vi "Initialize MeasurementLink Session.vi"(7 "remote connection options":T2, 8 "error in":errorcluster, 9 "initialize and close session behavior":T1, 10 "session initialization parameters":T3, 11 "session factory in":refnum<class "Session Factory.lvclass">) -> (0 "error out":errorcluster, 2 "session out":variant, 3 "session factory out":refnum<class "Session Factory.lvclass">)   [LabVIEW 2021, in "NI Session Management niDMM.lvlib" / "Session Factory.lvclass"]
uses:
  Session Factory.lvclass
  Instrument/ISession Factory/Session Initialization Parameters.ctl
  Instrument/ISession Factory/Remote Connection Options.ctl
  Instrument/ISession Factory/Initialize and Close Session Behavior.ctl
  Session Factory.lvclass/Session Factory.ctl
  Instrument/ISession Factory/ISession Factory.lvclass
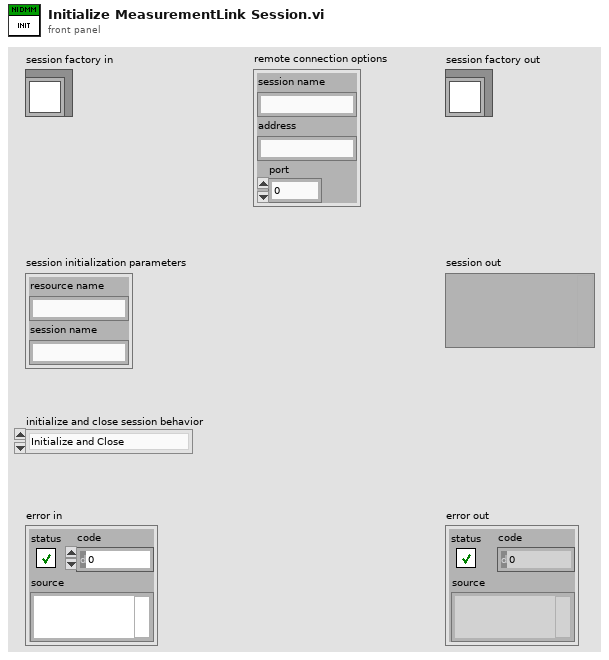
[diagram p1: front panel]
types:
  T1 = typedef "NI Session Management Instrument.lvlib/ISession Factory.lvclass/Initialize and Close Session Behavior.ctl" = enum16{"Initialize and Close", "Attach and Detach", "Initialize and Detach", "Attach and Close"}
  T2 = typedef "NI Session Management Instrument.lvlib/ISession Factory.lvclass/Remote Connection Options.ctl" = cluster{"session name":string, "address":string, "port":u32}
  T3 = typedef "NI Session Management Instrument.lvlib/ISession Factory.lvclass/Session Initialization Parameters.ctl" = cluster{"resource name":string, "session name":string}
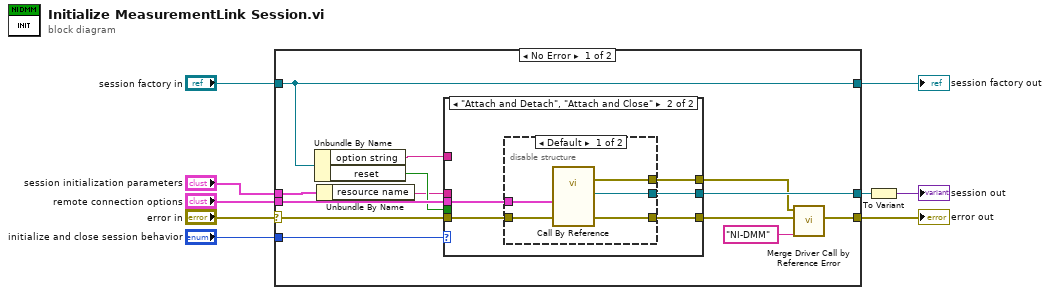
[diagram p0: block diagram]
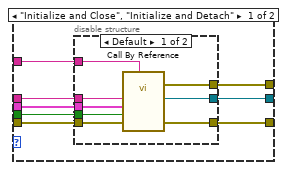
[diagram p2: hidden frame]
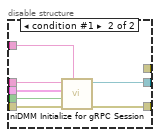
[diagram p3: hidden frame]
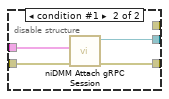
[diagram p4: hidden frame]
diagram:
  n1 = case shown="No Error" "error in" {
    selector: "error in" -> [w19 w60]
    tunnel: [w11 w60] -> w8
    tunnel: "session factory in" -> [w17 w61]
    tunnel: [w17 w61] -> w6
    tunnel: "initialize and close session behavior" -> [w22 _]
    tunnel: "remote connection options" -> [w21 _]
    tunnel: "session initialization parameters" -> [w18 _]
    tunnel: [w20 _] -> w2
    frame No Error {
      n2 = Unbundle By Name(w17) -> ("option string"=w16:string, "reset"=w15:bool)
      n3 = Unbundle By Name(w18) -> ("resource name"=w14:string)
      n4 = case shown="\"Attach and Detach\", \"Attach and Close\"" w22 {
        tunnel: w21 -> [w29 w50]
        tunnel: [w28 w49] -> w20
        tunnel: w19 -> [w30 w48]
        tunnel: [w27 w47] -> w12
        tunnel: w14 -> [w26 _]
        tunnel: w16 -> [w25 _]
        tunnel: w15 -> [w24 _]
        tunnel: [w23 w46] -> w10
        frame "Initialize and Close", "Initialize and Detach" {
          n5 = disable-structure shown="Default" {
            disable-tunnel: w30 -> [w38 w45]
            disable-tunnel: w29 -> [w37 w43]
            disable-tunnel: [w36 w40] -> w28
            disable-tunnel: [w35 w39] -> w27
            disable-tunnel: w26 -> [w34 w42]
            disable-tunnel: w25 -> [w33 w41]
            disable-tunnel: w24 -> [w32 w44]
            disable-tunnel: [w31 _] -> w23
            frame condition #0 (active) {
              n6 = call-by-ref "?"("Option String"=w33, "error in (no error)"=w38, "Reset Device"=w32, "gRPC Options"=w37, "Instrument Descriptor"=w34) -> (error out=w31:errorcluster, 0:"error out"=w35:errorcluster, "instrument handle out"=w36:refnum<k15>)  [unwired: 7 in, 1 out]
            }
            frame condition #1 {
              n7 = call <instrlib>:"niDMM Initialize for gRPC Session.vi"("Option String"=w41, "error in (no error)"=w45, "Reset Device"=w44, "gRPC Options"=w43, "Instrument Descriptor"=w42) -> ("error out"=w39:errorcluster, "instrument handle out"=w40:refnum<k15>)  [unwired: 5 in]
            }
          }
        }
        frame "Attach and Detach", "Attach and Close" {
          n8 = disable-structure shown="Default" {
            disable-tunnel: w50 -> [w55 w56]
            disable-tunnel: [w54 w57] -> w49
            disable-tunnel: w48 -> [w53 w59]
            disable-tunnel: [w52 w58] -> w47
            disable-tunnel: [w51 _] -> w46
            frame condition #0 (active) {
              n9 = call-by-ref "?"("error in (no error)"=w53, "gRPC Options"=w55) -> (error out=w51:errorcluster, 0:"error out"=w52:errorcluster, "instrument handle out"=w54:refnum<k15>)  [unwired: 10 in, 1 out]
            }
            frame condition #1 {
              n10 = call <instrlib>:"niDMM Attach gRPC Session.vi"("error in (no error)"=w59, "gRPC Options"=w56) -> ("error out"=w58:errorcluster, "instrument handle out"=w57:refnum<k15>)  [unwired: 8 in]
            }
          }
        }
      }
      n11 = call "Merge Driver Call by Reference Error.vi"("driver name"="NI-DMM", "called vi error"=w12, "call by ref error"=w10) -> ("error out"=w11:errorcluster)  [unwired: 8 in]
    }
    frame Error {
    }
  }
  "error out" <- w8
  "session factory out" <- w6
  n12 = To Variant(anything=w2) -> (Variant=→"session out":variant)
